vi "_builtins_has_selection.vi"(8 "error in (no error)":errorcluster, 10 "Focus":enum8{"FP", "BD"}(ring), 11 "VI Refnum in":refnum<vi>) -> (0 "error out":errorcluster, 1 "size":i32, 2 "SelList[]":refnum<vi>[](array[refnum]), 3 "VI Refnum out":refnum<vi>)   [LabVIEW 2019, in "Script.lvlib"]
doc: "Returns the Selection List of GObjects on the Panel or Diagram.\n\nCreated by: Ryan Pacini"
uses:
  Script.lvlib
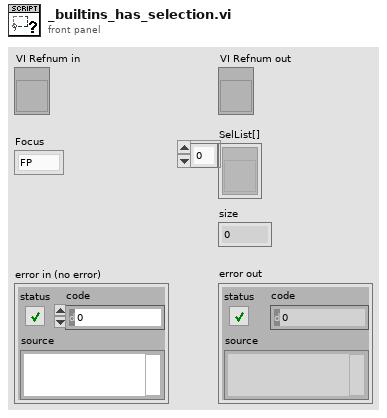
[diagram p1: front panel]
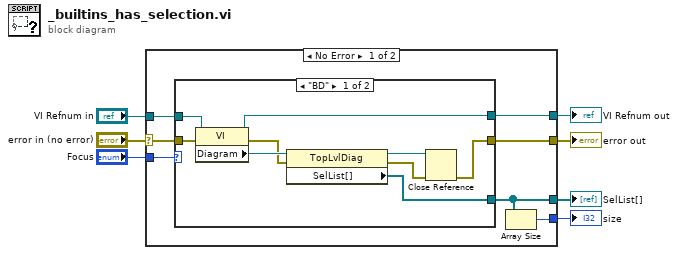
[diagram p0: block diagram]
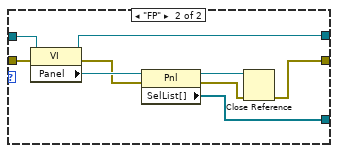
[diagram p2: hidden frame]
diagram:
  n1 = case shown="No Error" "error in (no error)" {
    selector: "error in (no error)" -> [w13 w33]
    tunnel: "Focus" -> [w10 _]
    tunnel: "VI Refnum in" -> [w14 w34]
    tunnel: [w12 w33] -> w4
    tunnel: [w11 w34] -> w3
    tunnel: [w9 _] -> w2
    tunnel: [w8 _] -> w1
    frame No Error {
      n2 = case shown="\"BD\"" w10 {
        tunnel: w14 -> [w23 w32]
        tunnel: w13 -> [w22 w31]
        tunnel: [w21 w30] -> w12
        tunnel: [w20 w29] -> w11
        tunnel: [w15 w24] -> w9
        frame "BD" {
          n3 = property class="VI"(reference=w23, error in=w22) -> (reference out=w20:refnum<vi>, error out=w18:errorcluster, "Diagram"=w19:refnum<vi>)
          n4 = property class="TopLvlDiag"(reference=w19, error in=w18) -> (reference out=w16:refnum<vi>, error out=w17:errorcluster, "SelList[]"=w15:refnum<vi>[])
          n5 = Close Reference(reference=w16, error in (no error)=w17) -> (error out=w21:errorcluster)
        }
        frame "FP" {
          n6 = property class="VI"(reference=w32, error in=w31) -> (reference out=w29:refnum<vi>, error out=w27:errorcluster, "Panel"=w28:refnum<vi>)
          n7 = property class="Pnl"(reference=w28, error in=w27) -> (reference out=w25:refnum<vi>, error out=w26:errorcluster, "SelList[]"=w24:refnum<vi>[])
          n8 = Close Reference(reference=w25, error in (no error)=w26) -> (error out=w30:errorcluster)
        }
      }
      n9 = Array Size(array=w9) -> (size(s)=w8:i32)
    }
    frame Error {
    }
  }
  "VI Refnum out" <- w3
  "error out" <- w4
  "SelList[]" <- w2
  "size" <- w1
